vi "Wait for Operation Complete.vi"(8 "error in (no error)":errorcluster, 9 "Maximum Time (10000ms)":u32=10000, 11 "VISA resource name":refnum<visa-resource-name>) -> (0 "error out":errorcluster, 3 "VISA resource name out":refnum<visa-resource-name>)   [LabVIEW 2013, in "Tektronix DPO MSO 2000 4000 Series.lvlib"]
doc: "This VI waits for the instrument to complete the execution of all pending operations. The <B>Timeout</B> control specifies the maximum time to wait for operation complete in milliseconds."
uses:
  Tektronix DPO MSO 2000 4000 Series.lvlib
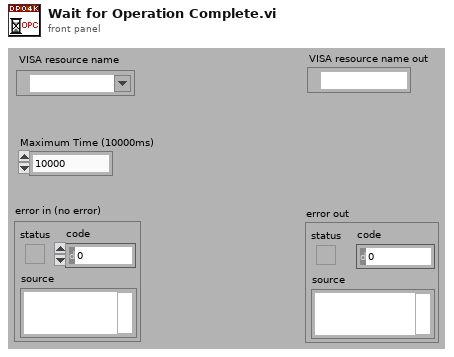
[diagram p1: front panel]
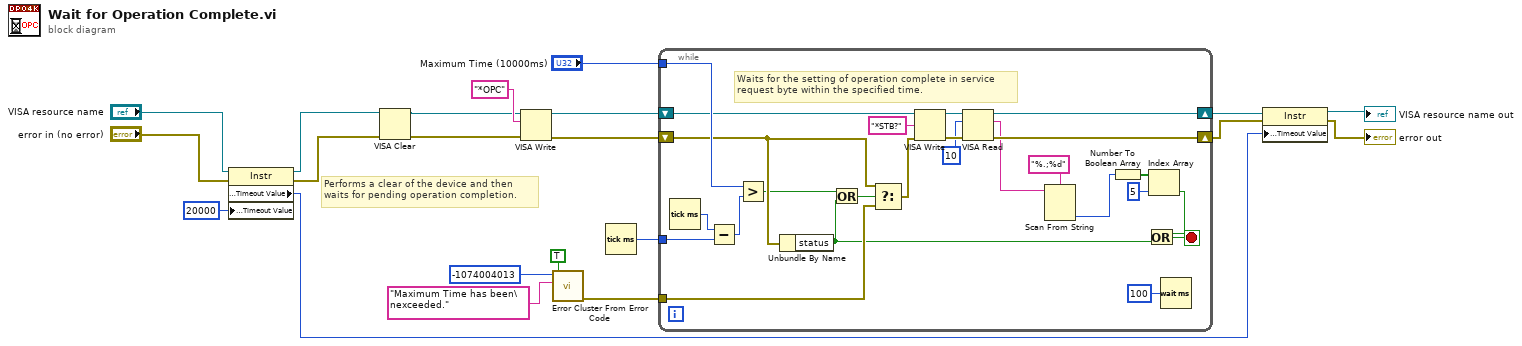
[diagram p0: block diagram]
diagram:
  # "Performs a clear of the device and then\nwaits for pending operation completion."
  n1 = property class="Instr"(reference="VISA resource name", error in="error in (no error)", "General Settings:Timeout Value"=u32 20000) -> (reference out=w12:refnum<visa-resource-name>, error out=w11:errorcluster, "General Settings:Timeout Value"=w9:u32)
  n2 = VISA Clear(VISA resource name=w12, error in (no error)=w11) -> (VISA resource name out=w2:refnum<visa-resource-name>, error out=w1:errorcluster)
  n3 = VISA Write(VISA resource name=w2, write buffer="*OPC", error in (no error)=w1) -> (VISA resource name out=w18:refnum<visa-resource-name>, error out=w17:errorcluster)  [unwired: 1 out]
  n4 = call <vilib>:"Error Cluster From Error Code.vi"("show call chain? (False)"=TRUE, "error message (\"\")"="Maximum Time has been\nexceeded." ("error message (\"\")"), "error code (0)"=-1074004013) -> ("error out"=w16:errorcluster)  [unwired: 6 in]
  n5 = Tick Count (ms)() -> (millisecond timer value=w20:u32)
  n6 = while {
    tunnel: w20 -> [w43]
    tunnel: "Maximum Time (10000ms)" -> [w41]
    shift-right: [w26] -> w8
    shift-left: w18 -> [w32]
    shift-right: [w25] -> w7
    shift-left: w17 -> [w38]
    tunnel: w16 -> [w39]
    stop <- w37 stop-if-true
    # "Waits for the setting of operation complete in service\nrequest byte within the specified time."
    n7 = Tick Count (ms)() -> (millisecond timer value=w44:u32)
    n8 = Subtract(x=w44, y=w43) -> (x-y=w42:u32)
    n9 = Greater?(x=w41, y=w42) -> (0:w35:bool)
    n10 = Unbundle By Name(w38) -> ("status"=w34:bool)
    n11 = Or(x=w35, y=w34) -> (x .or. y?=w40:bool)
    n12 = Select(t=w38, s=w40, f=w39) -> (s? t:f=w33:errorcluster)
    n13 = VISA Write(VISA resource name=w32, write buffer="*STB?", error in (no error)=w33) -> (VISA resource name out=w28:refnum<visa-resource-name>, error out=w29:errorcluster)  [unwired: 1 out]
    n14 = VISA Read(VISA resource name=w28, byte count=u32 10, error in (no error)=w29) -> (VISA resource name out=w26:refnum<visa-resource-name>, read buffer=w23:string, error out=w25:errorcluster)  [unwired: 1 out]
    n15 = Scan From String(format string="%.;%d", input string=w23) -> (output 1=w24:i32)  [unwired: 3 in, 3 out]
    n16 = Number To Boolean Array(number=w24) -> (Boolean array=w46:bool[])
    n17 = Index Array(array=w46, index=5) -> (element=w36:bool)
    n18 = Or(x=w36, y=w34) -> (x .or. y?=w37:bool)
    n19 = Wait (ms)(milliseconds to wait=u32 100) -> ()  [unwired: 1 out]
  }
  n20 = property class="Instr"(reference=w8, error in=w7, "General Settings:Timeout Value"=w9) -> (reference out=→"VISA resource name out":refnum<visa-resource-name>, error out=→"error out":errorcluster)
